vi "Get Initialized.vi"(8 "error in (no error)":errorcluster, 11 "Panel in":refnum<class "Panel.lvclass">) -> (0 "error out":errorcluster, 2 "Initialized":bool, 3 "Panel out":refnum<class "Panel.lvclass">)   [LabVIEW 2014, in "OOPanel.lvlib" / "Panel.lvclass"]
uses:
  Panel.lvclass
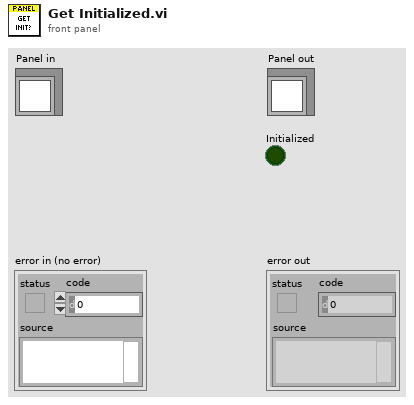
[diagram p1: front panel]
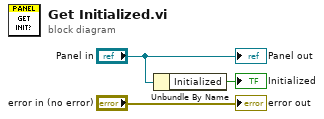
[diagram p0: block diagram]
diagram:
  n1 = Unbundle By Name("Panel in") -> ("Initialized"=→"Initialized":bool)
  "error out" <- "error in (no error)"
  "Panel out" <- "Panel in"
